vi "Write Invidual Beams.vi"(8 "error in (no error)":errorcluster, 10 "Invidual Beams":u8[][](array[numeric])=[[0, 0], [64, 0], [32, 0], [16, 0], [8, 0], [4, 0], [2, 0], [1, 0], [0, 64], [0, 32], [0, 16], [0, 8], [0, 4], [0, 2], [0, 1]] format="%x", 11 "Toggle 8 in":refnum<class "Toggle 8.lvclass">) -> (0 "error out":errorcluster, 3 "Toggle 8 out":refnum<class "Toggle 8.lvclass">)   [LabVIEW 2020, in "Toggle 8.lvclass"]
uses:
  Toggle 8.lvclass
  Toggle 8.lvclass/Toggle 8.ctl
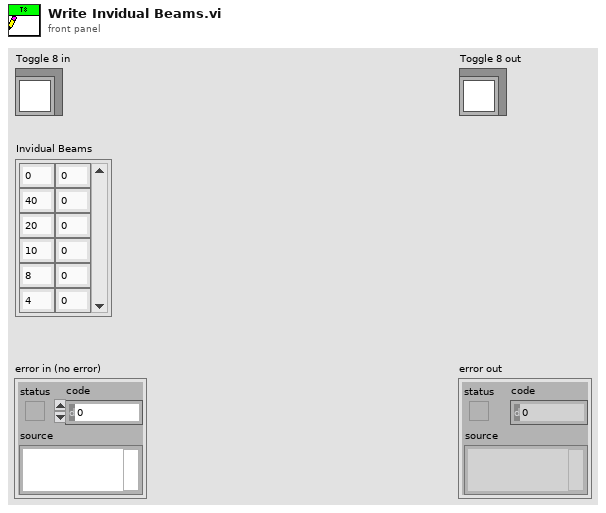
[diagram p1: front panel]
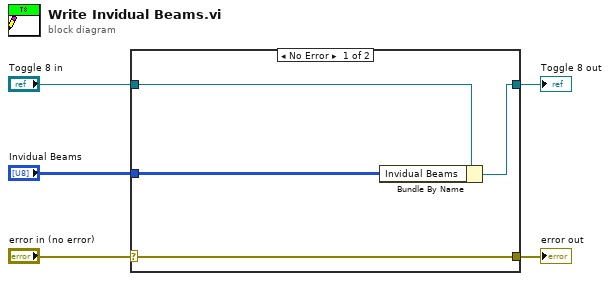
[diagram p0: block diagram]
diagram:
  n1 = case shown="No Error" "error in (no error)" {
    selector: "error in (no error)" -> [w9 w10]
    tunnel: [w9 w10] -> w4
    tunnel: [w7 w11] -> w2
    tunnel: "Toggle 8 in" -> [w8 w11]
    tunnel: "Invidual Beams" -> [w6 _]
    frame No Error {
      n2 = Bundle By Name(cluster=w8, "Invidual Beams"=w6) -> (w7:refnum<class "Toggle 8.lvclass">)
    }
    frame Error {
    }
  }
  "error out" <- w4
  "Toggle 8 out" <- w2
